vi "吸光值计算.vi"(3 "吸光值算法":enum16{"对数", "减法"}(ring), 6 "F1":dbl, 7 "F0":dbl) -> (1 "测量吸光度":dbl)   [LabVIEW 2016, in "曲线模型.xctl"]
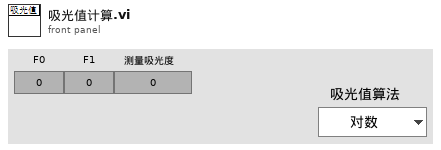
[diagram p1: front panel]
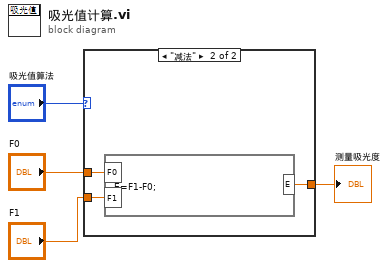
[diagram p0: block diagram]
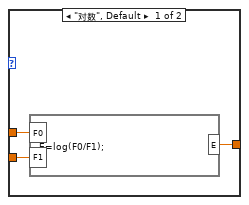
[diagram p2: hidden frame]
diagram:
  n1 = case shown="\"减法\"" "吸光值算法" {
    tunnel: "F0" -> [w7 w10]
    tunnel: "F1" -> [w6 w9]
    tunnel: [w5 w8] -> w2
    frame "对数", Default {
      n2 = formula code="E=log(F0/F1);"("F0"=w7, "F1"=w6) -> ("E"=w5:dbl)
    }
    frame "减法" {
      n3 = formula code="E=F1-F0;"("F0"=w10, "F1"=w9) -> ("E"=w8:dbl)
    }
  }
  "测量吸光度" <- w2
